vi "NewCore.vi"(8 "error in (no error)":errorcluster, 10 "ParamsArray":variant[](array[variant]), 11 "RoomWithBomb":refnum<class "RoomWithBomb.lvclass">) -> (0 "error out":errorcluster, 3 "RoomWithBomb":refnum<class "RoomWithBomb.lvclass">)   [LabVIEW 2020, in "RoomWithBomb.lvclass"]
uses:
  RoomWithBomb.lvclass
  Private/TypeDef/privateData.ctl
  TypeDef/RoomWithBombParams.ctl
  RoomWithBomb.lvclass/RoomWithBomb.ctl
  Room/Room.lvclass
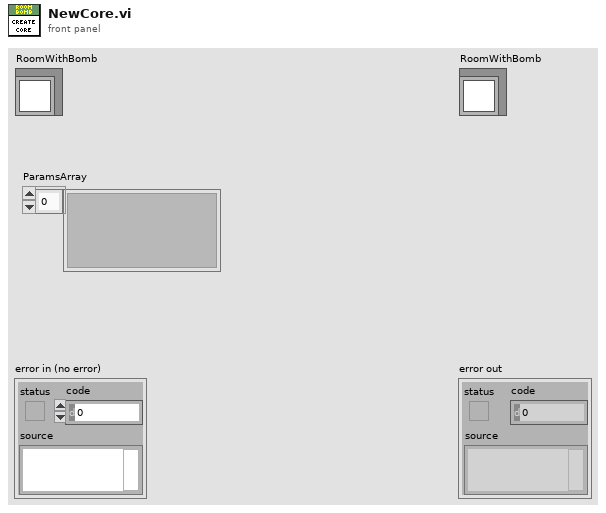
[diagram p1: front panel]
types:
  T1 = typedef "RoomWithBomb.lvclass/RoomWithBombParams.ctl" = cluster{"bomb":bool}
  T2 = typedef "RoomWithBomb.lvclass/privateData.ctl" = cluster{"bomb":bool}
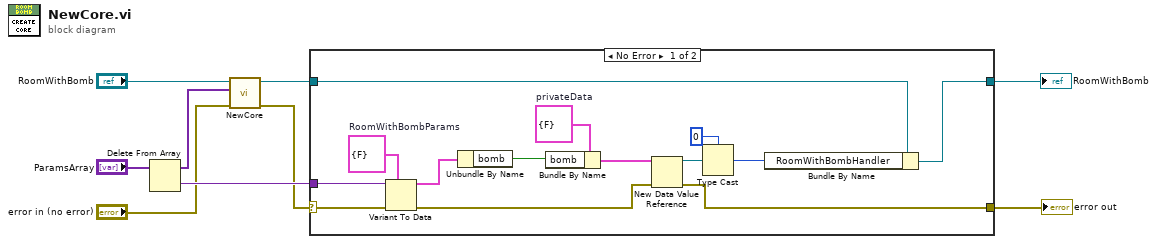
[diagram p0: block diagram]
diagram:
  n1 = Delete From Array(array="ParamsArray") -> (deleted portion=w4:variant, array with subset deleted=w3:variant[])  [unwired: 2 in]
  n2 = call-parent "NewCore.vi"("error in (no error)"="error in (no error)", "ParamsArray"=w3, "Room"="RoomWithBomb") -> ("error out"=w2:errorcluster, "Room"=w9:refnum<class "RoomWithBomb.lvclass">)  [unwired: 7 in]
  n3 = case shown="No Error" w2 {
    selector: w2 -> [w12 w25]
    tunnel: [w16 w25] -> w7
    tunnel: [w18 w24] -> w8
    tunnel: w9 -> [w17 w24]
    tunnel: w4 -> [w10 _]
    frame No Error {
      w14 = T1 {"bomb"=FALSE}  # RoomWithBombParams
      w20 = T2 {"bomb"=FALSE}  # privateData
      n4 = Variant To Data(error in=w12, type=w14, Variant=w10) -> (data=w13:T1, error out=w11:errorcluster)
      n5 = Unbundle By Name(w13) -> ("bomb"=w15:bool)
      n6 = Bundle By Name(cluster=w20, "bomb"=w15) -> (w19:T2)
      n7 = New Data Value Reference(data value=w19, error in=w11) -> (data value reference=w23:refnum<data-value>, error out=w16:errorcluster)
      n8 = Type Cast(type=u32 0, x=w23) -> (*(type *) &x=w21:u32)
      n9 = Bundle By Name(cluster=w17, "RoomWithBombHandler"=w21) -> (w18:refnum<class "RoomWithBomb.lvclass">)
    }
    frame Error {
    }
  }
  "error out" <- w7
  "RoomWithBomb" <- w8
